vi "Gasflaschen Info.vi"(11 "Gasflasche MFC2":T1 items=["----"=10000, "IAG NH3 3000"=0, "IAG NH3 200"=1, "IAG NH3 2000"=2, "IAG MG"=3, "IAG O2"=4]) -> (1 "String":string, 2 "Konzentration IST":dbl, 3 "Chargennummer":string, 4 "Einheitindex":i32, 5 "Component":i32, 7 "Component found":bool)   [LabVIEW 2020, in "EPA 1065.lvlib" / "HovaCAL Interference verificaton.lvlib"]
uses:
  HovaCAL Interference verificaton.lvlib
  Seiten/System Einstellungen V2/System Einstellungen V2.lvlib
  Seiten/System Einstellungen V2/Aktion FGV Gasbottledefinition.ctl
  Linearisierung V2/SpanEinstellungen/SpanEinstellungen.lvlib
  Seiten/System Einstellungen V2/Gasflasche Auswahl.ctl
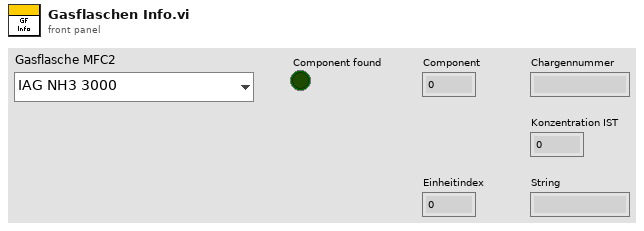
[diagram p1: front panel]
types:
  T1 = typedef "System Einstellungen V2.lvlib/Gasflasche Auswahl.ctl" = u16
  T2 = typedef "System Einstellungen V2.lvlib/Aktion FGV Gasbottledefinition.ctl" = enum16{"lesen", "schreiben", "löschen", "laden", "speichern", "exportieren", "importieren"}
  T3 = typedef "System Einstellungen V2.lvlib/Gasflasche gesamt.ctl" = cluster{"Gasflasche":T4, "Trägergas":T5, "Komponenten":T6[]}
  T4 = typedef "System Einstellungen V2.lvlib/Gasflasche.ctl" = cluster{"Gasname für die Auswahl":string, "Chargennummer":string, "Ablaufdatum":timestamp}
  T5 = typedef "System Einstellungen V2.lvlib/Traegergas.ctl" = string
  T6 = typedef "System Einstellungen V2.lvlib/Gasflaschenkomponente.ctl" = cluster{"Gasauswahl":string, "Konzentration IST":dbl, "Einheit":string, "Genauigkeit":dbl}
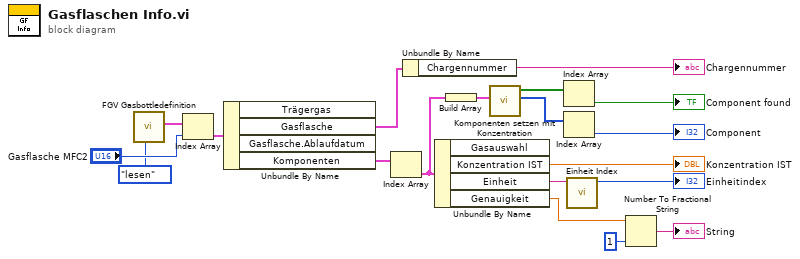
[diagram p0: block diagram]
diagram:
  n1 = call "FGV Gasbottledefinition.vi"("Aktion"=Aktion_FGV_Gasbottledefinition."lesen") -> ("Gasflaschen Liste gesamt"=w4:T3[])  [unwired: 8 in, 2 out]
  n2 = Index Array(array=w4, index="Gasflasche MFC2") -> (element=w3:T3)
  n3 = Unbundle By Name(w3) -> ("Gasflasche"=w12:T4, "Komponenten"=w7:T6[])  [unwired: 2 out]
  n4 = Index Array(array=w7) -> (element=w8:T6)  [unwired: 1 in]
  n5 = Unbundle By Name(w12) -> ("Chargennummer"=→"Chargennummer":string)
  n6 = Unbundle By Name(w8) -> ("Konzentration IST"=→"Konzentration IST":dbl, "Einheit"=w15:string, "Genauigkeit"=w17:dbl)  [unwired: 1 out]
  n7 = Build Array(w8) -> (w9:T6[])
  n8 = call "Komponenten setzen mit Konzentration.vi"("Komponenten"=w9) -> ("Index"=w11:i32[], "found"=w10:bool[])  [unwired: 6 in, 3 out]
  n9 = Index Array(array=w10) -> (element=→"Component found":bool)  [unwired: 1 in]
  n10 = Index Array(array=w11) -> (element=→"Component":i32)  [unwired: 1 in]
  n11 = call "Einheit Index.vi"("Einheit in String"=w15) -> ("Elementindex"=→"Einheitindex":i32)  [unwired: 10 in]
  n12 = Number To Fractional String(number=w17, precision (6)=i16 1 ("Genauigkeit (6)")) -> (F-format string=→"String":string)  [unwired: 2 in]
